vi "List Triggers.vi"(8 "error in (no error)":errorcluster, 11 "NI DMM Driver in":refnum<class "DMM.NI.lvclass">) -> (0 "error out":errorcluster, 2 "Trigger Names":string[](array[string]), 3 "NI DMM Driver out":refnum<class "DMM.NI.lvclass">)   [LabVIEW 2020, in "NI DMM Driver.lvlib" / "DMM.NI.lvclass"]
doc: "List the triggers supported by the DMM Driver."
uses:
  DMM.NI.lvclass
  <instrlib>/niDMM/nidmm.llb/niDMM Sample Trigger.ctl
panel:
  in  "Sample Trigger":T1
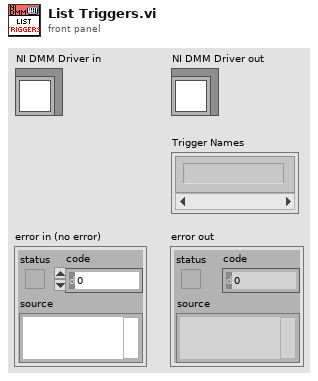
[diagram p1: front panel]
types:
  T1 = typedef "niDMM Sample Trigger.ctl" = enum16{"Immediate", "External", "TTL 0", "TTL 1", "TTL 2", "TTL 3", "TTL 4", "TTL 5", "TTL 6", "Interval", "Software", "TTL 7", "PXI Star", "LBR Trig 1", "Aux Trig 1"}
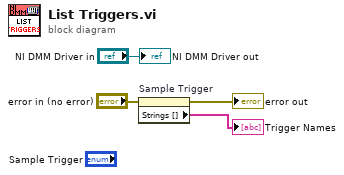
[diagram p0: block diagram]
diagram:
  n1 = property on="Sample Trigger" class="Enum (strict)"(error in="error in (no error)") -> (error out=→"error out":errorcluster, "Strings []"=→"Trigger Names":string[])  [unwired: 1 in, 1 out]
  "NI DMM Driver out" <- "NI DMM Driver in"
